vi "LEIN node ID.vi"() -> ()   [LabVIEW 2010]
panel:
  out "ID":T1 {"LEIN impl. code" format="%.0x"}
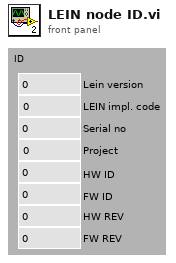
[diagram p1: front panel]
types:
  T1 = cluster{"Lein version":u8, "LEIN impl. code":u8, "Serial no":u16, "Project":u16, "HW ID":u8, "FW ID":u8, "HW REV":u8, "FW REV":u8}
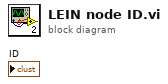
[diagram p0: block diagram]
diagram:
